vi "Close Hologram Engine.vi"(8 "error in (no error)":errorcluster) -> ()   [LabVIEW 2020]
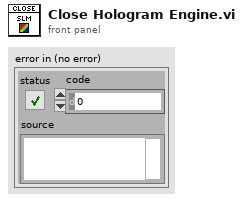
[diagram p1: front panel]
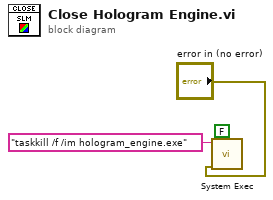
[diagram p0: block diagram]
diagram:
  n1 = call <vilib>:"System Exec.vi"("wait until completion? (T)"=FALSE, "error in (no error)"="error in (no error)", "command line"="taskkill /f /im hologram_engine.exe") -> ()  [unwired: 5 in, 4 out]
